vi "Check Date Format.vi"(8 "error in (no error)":errorcluster, 11 "Date":string) -> (0 "error out":errorcluster, 3 "Format?":bool)   [LabVIEW 2021, in "User Interface.lvlib"]
uses:
  User Interface.lvlib
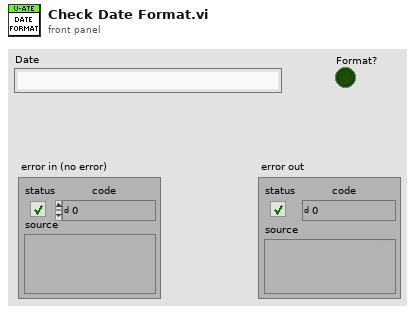
[diagram p1: front panel]
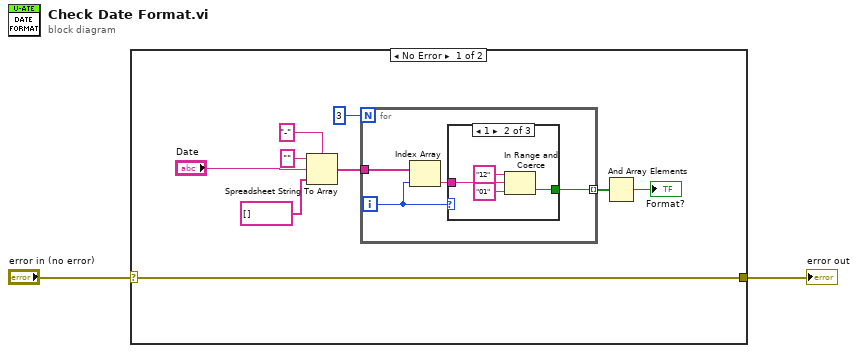
[diagram p0: block diagram]
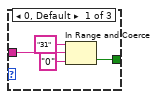
[diagram p2: hidden frame]
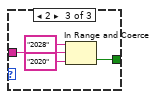
[diagram p3: hidden frame]
diagram:
  n1 = case shown="No Error" "error in (no error)" {
    selector: "error in (no error)" -> [w3 w28]
    tunnel: [w3 w28] -> w1
    frame No Error {
      n2 = Spreadsheet String To Array(delimiter (Tab)="-", format string="", spreadsheet string="Date", array type (2D Dbl)=string[] []) -> (array=w11:string[])
      n3 = for {
        N: 3 -> [_]
        tunnel: w11 -> [w15]
        tunnel: [w12] -> w10 mode=indexing
        i -> [w14]
        n4 = Index Array(array=w15, index=w14) -> (element=w13:string)
        n5 = case shown="1" w14 {
          tunnel: w13 -> [w19 w23 w27]
          tunnel: [w16 w20 w24] -> w12
          frame 0, Default {
            n6 = In Range and Coerce(upper limit="31", x=w19, lower limit="0") -> (In Range?=w16:bool)  [unwired: 1 out]
          }
          frame 1 {
            n7 = In Range and Coerce(upper limit="12", x=w23, lower limit="01") -> (In Range?=w20:bool)  [unwired: 1 out]
          }
          frame 2 {
            n8 = In Range and Coerce(upper limit="2028", x=w27, lower limit="2020") -> (In Range?=w24:bool)  [unwired: 1 out]
          }
        }
      }
      n9 = And Array Elements(Boolean array=w10) -> (logical AND=→"Format?":bool)
    }
    frame Error {
    }
  }
  "error out" <- w1
